vi "Labvıew aviyonik.vi"() -> ()   [LabVIEW 2019]
uses:
  <vilib>/Instr/_visa.llb/VISA Configure Serial Port (Instr).vi
panel:
  out "decimal integer string":string
  out "VERİ GÖZLEM":string="22.63 72.45\r\n"
  in  "DATALARI KAYDETMEK ICIN DOSYA SECINIZ":path
  out "SISTEM DURUM":string
  out "?":bool
  in  "IRTIFA ALT  LIMIT":dbl
  in  "IRTIFA UST LIMIT":dbl
  in  "X ALT  LIMIT":dbl
  in  "X UST LIMIT":dbl
  out "Y":dbl(slide) scale=0.0..90.0
  out "X":dbl(slide) scale=0.0..90.0
  out "X ESEN IVME":dbl
  out "IVME":dbl(knob) scale=0.0..1.0
  out "Y ACISI":dbl
  out "X ACISI":dbl
  in  "?":bool
  in  "SERİ PORT":refnum<visa-resource-name>="COM3"
  out "IRTIFA":dbl=0.7199999999720603
  out "BASINC hPa":dbl
  out "BASINC":dbl(knob) scale=0.0..5000.0
  out "IRTIFA":dbl(slide) scale=0.0..1000.0
  out "SICAKLIK °C":dbl=22.0
  out "SICAKLIK":dbl(slide) scale=0.0..100.0
  # "SISTEM TEST"
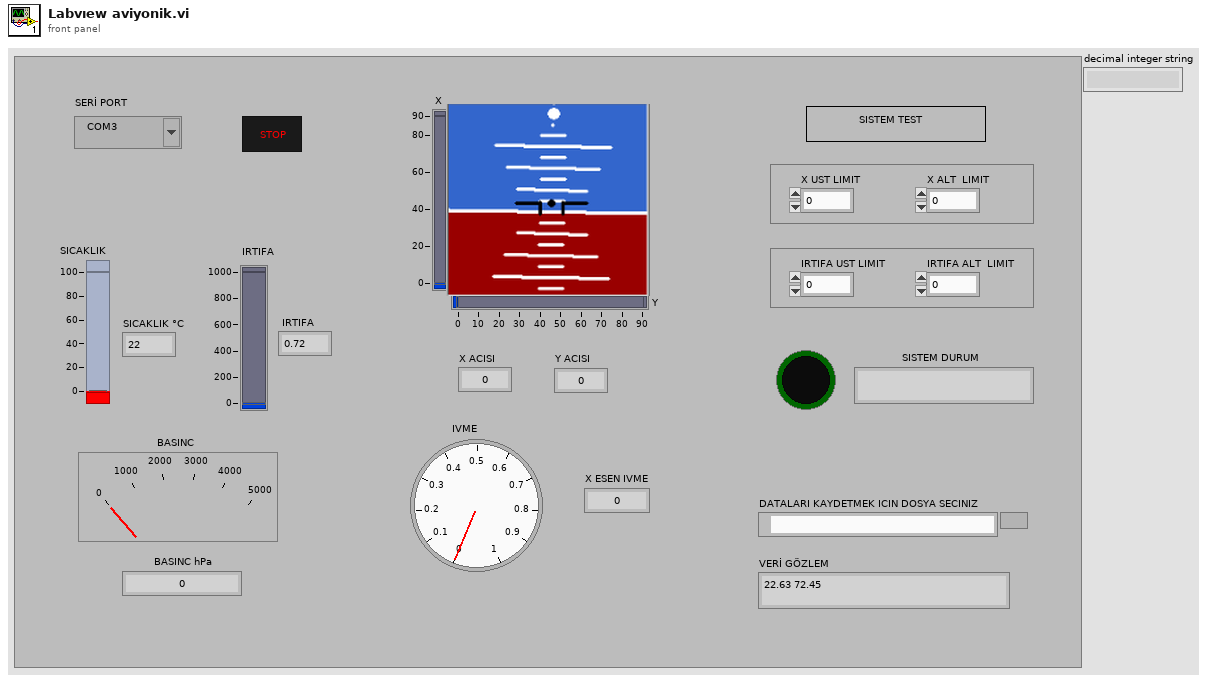
[diagram p1: front panel]
types:
  T1 = enum16{"open", "replace", "create", "open or create", "replace or create", "replace or create with confirmation"}
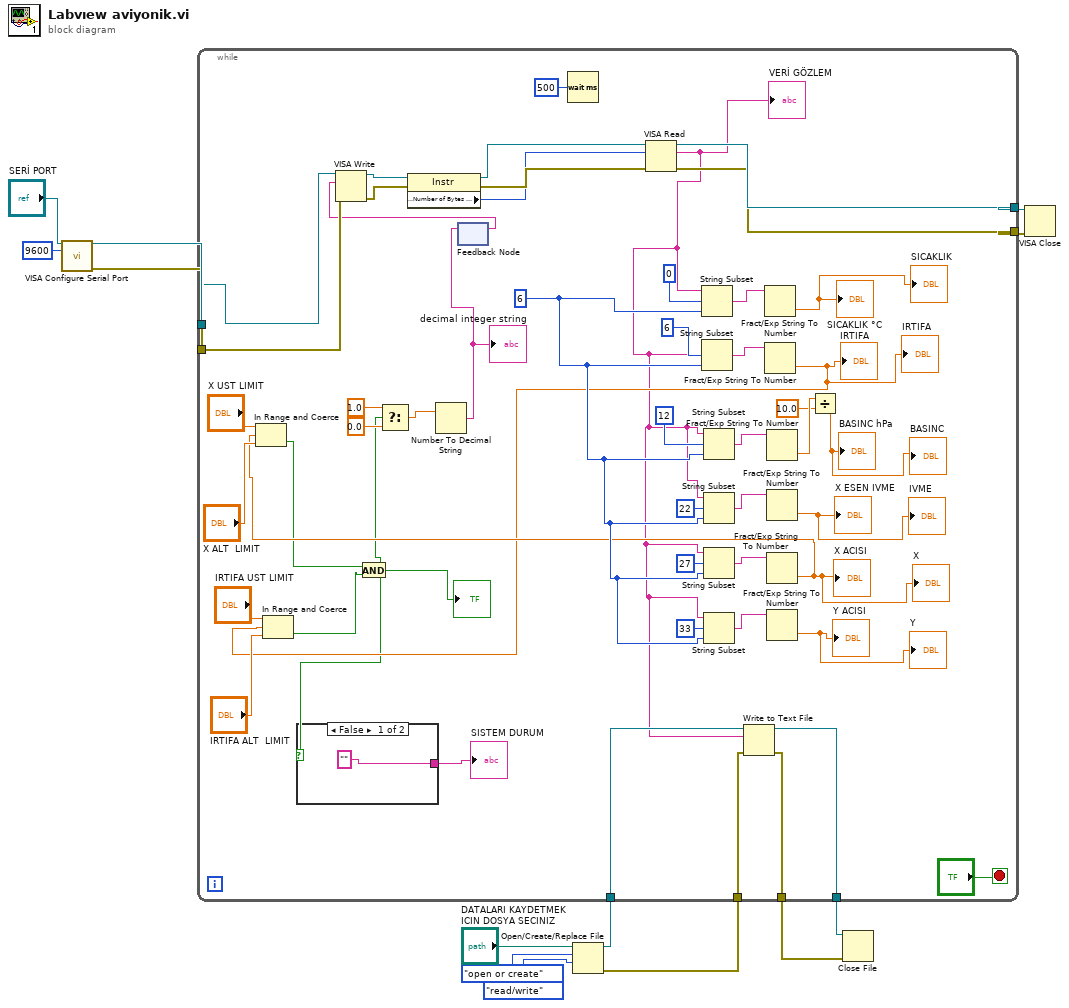
[diagram p0: block diagram]
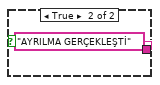
[diagram p2: hidden frame]
diagram:
  n1 = call-poly "VISA Configure Serial Port"("VISA resource name"="SERİ PORT", "baud rate (9600)"=u32 9600) -> ("VISA resource name out"=w12:refnum<visa-resource-name>, "error out"=w11:errorcluster)  [unwired: 12 in]
  n2 = Open/Create/Replace File(file path (use dialog)="DATALARI KAYDETMEK ICIN DOSYA SECINIZ", operation (0:open)=T1."open or create", access (0:read/write)=enum16{"read/write", "read-only", "write-only"}."read/write") -> (refnum out=w4:refnum<file>, error out=w1:errorcluster)  [unwired: 3 in, 1 out]
  n3 = while {
    tunnel: w12 -> [w38]
    tunnel: w11 -> [w61]
    tunnel: [w57] -> w10
    tunnel: [w56] -> w9
    tunnel: w4 -> [w18]
    tunnel: [w17] -> w3
    tunnel: [w16] -> w2
    tunnel: w1 -> [w15]
    stop <- "?" stop-if-true
    w32 = 6 ("length (rest)")
    n4 = feedback #1() -> (w34:string)  [unwired: 1 in]
    n5 = VISA Write(VISA resource name=w38, write buffer=w34, error in (no error)=w61) -> (VISA resource name out=w63:refnum<visa-resource-name>, error out=w62:errorcluster)  [unwired: 1 out]
    n6 = property class="Instr"(reference=w63, error in=w62) -> (reference out=w60:refnum<visa-resource-name>, error out=w59:errorcluster, "Serial Settings:Number of Bytes at Serial Port"=w58:u32)
    n7 = Wait (ms)(milliseconds to wait=u32 500) -> ()  [unwired: 1 out]
    n8 = VISA Read(VISA resource name=w60, byte count=w58, error in (no error)=w59) -> (VISA resource name out=w57:refnum<visa-resource-name>, read buffer=w14:string, error out=w56:errorcluster)  [unwired: 1 out]
    "VERİ GÖZLEM" <- w14
    n9 = String Subset(string=w14, offset (0)=0, length (rest)=w32) -> (substring=w52:string)
    n10 = String Subset(string=w14, offset (0)=6, length (rest)=w32) -> (substring=w51:string)
    n11 = String Subset(string=w14, offset (0)=12, length (rest)=w32) -> (substring=w46:string)
    n12 = String Subset(string=w14, offset (0)=22, length (rest)=w32) -> (substring=w45:string)
    n13 = String Subset(string=w14, offset (0)=27, length (rest)=w32) -> (substring=w44:string)
    n14 = String Subset(string=w14, offset (0)=33, length (rest)=w32) -> (substring=w43:string)
    n15 = Write to Text File(file (use dialog)=w18, text=w14, error in=w15) -> (refnum out=w17:refnum<file>, error out=w16:errorcluster)  [unwired: 1 in, 1 out]
    n16 = Fract/Exp String To Number(string=w52) -> (number=→"SICAKLIK °C" →"SICAKLIK":dbl)  [unwired: 3 in, 1 out]
    n17 = Fract/Exp String To Number(string=w51) -> (number=w21:dbl)  [unwired: 3 in, 1 out]
    "IRTIFA" <- w21
    "IRTIFA" <- w21
    n18 = In Range and Coerce(upper limit="IRTIFA UST LIMIT", x=w21, lower limit="IRTIFA ALT  LIMIT") -> (In Range?=w22:bool)  [unwired: 1 out]
    n19 = Fract/Exp String To Number(string=w46) -> (number=w40:dbl)  [unwired: 3 in, 1 out]
    n20 = Fract/Exp String To Number(string=w45) -> (number=→"X ESEN IVME" →"IVME":dbl)  [unwired: 3 in, 1 out]
    n21 = Fract/Exp String To Number(string=w44) -> (number=w27:dbl)  [unwired: 3 in, 1 out]
    "X ACISI" <- w27
    "X" <- w27
    n22 = In Range and Coerce(upper limit="X UST LIMIT", x=w27, lower limit="X ALT  LIMIT") -> (In Range?=w23:bool)  [unwired: 1 out]
    n23 = And(x=w23, y=w22) -> (x .and. y?=w20:bool)
    "?" <- w20
    n24 = case shown="False" w20 {
      tunnel: ["" "AYRILMA GERÇEKLEŞTİ" ("String")] -> w19
      frame False {
      }
      frame True {
      }
    }
    "SISTEM DURUM" <- w19
    n25 = Select(t=1.0, s=w20, f=0.0) -> (s? t:f=w37:dbl)
    n26 = Number To Decimal String(number=w37) -> (decimal integer string=w35:string)  [unwired: 1 in]
    "decimal integer string" <- w35
    n27 = feedback-in #1(w35) -> ()
    n28 = Fract/Exp String To Number(string=w43) -> (number=→"Y ACISI" →"Y":dbl)  [unwired: 3 in, 1 out]
    n29 = Divide(x=w40, y=10.0) -> (x/y=→"BASINC hPa" →"BASINC":dbl)
  }
  n30 = Close File(refnum=w3, error in=w2) -> ()  [unwired: 2 out]
  n31 = VISA Close(VISA resource name=w10, error in (no error)=w9) -> ()  [unwired: 1 out]
